vi "Store Active Guidance.vi"(8 "error in (no error)":errorcluster, 10 "Guidance In":refnum<class "Guidance.lvclass">, 11 "Vessel in":refnum<class "Vessel.lvclass">) -> (0 "error out":errorcluster, 3 "Vessel out":refnum<class "Vessel.lvclass">)   [LabVIEW 2014, in "Vessel.lvclass"]
uses:
  Vessel.lvclass
  Guidance/Guidance.lvclass
  Vessel.lvclass/Vessel.ctl
  Supervisor/Supervisor.lvclass
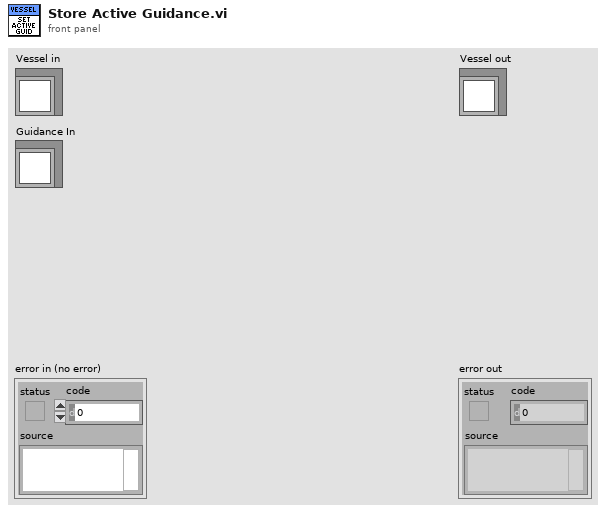
[diagram p1: front panel]
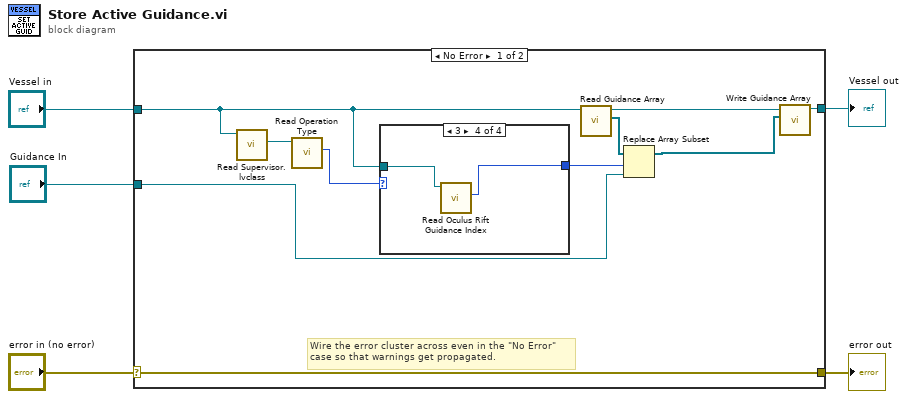
[diagram p0: block diagram]
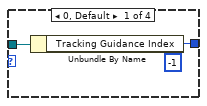
[diagram p2: hidden frame]
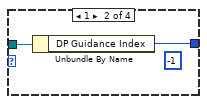
[diagram p3: hidden frame]
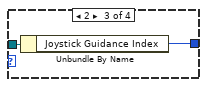
[diagram p4: hidden frame]
diagram:
  n1 = case shown="No Error" "error in (no error)" {
    selector: "error in (no error)" -> [w15 w25]
    tunnel: [w15 w25] -> w4
    tunnel: [w10 w24] -> w2
    tunnel: "Vessel in" -> [w11 w24]
    tunnel: "Guidance In" -> [w7 _]
    frame No Error {
      # "Wire the error cluster across even in the \"No Error\"\ncase so that warnings get propagated."
      n2 = call "Read Supervisor.lvclass.vi"("Vessel in"=w11) -> ("Supervisor.lvclass"=w14:refnum<class "Supervisor.lvclass">)  [unwired: 8 in, 2 out]
      n3 = call-dynamic "Read Operation Type.vi"("Supervisor in"=w14) -> ("Operation Type"=w13:u16)  [unwired: 8 in, 2 out]
      n4 = case shown="3" w13 {
        tunnel: w11 -> [w17 w19 w21 w23]
        tunnel: [w16 w18 w20 w22] -> w8
        frame 0, Default {
          (unwired) -1 ("DP Guidance Index")
          n5 = Unbundle By Name(w17) -> ("Tracking Guidance Index"=w16:i32)
        }
        frame 1 {
          (unwired) -1 ("DP Guidance Index")
          n6 = Unbundle By Name(w19) -> ("DP Guidance Index"=w18:i32)
        }
        frame 2 {
          n7 = Unbundle By Name(w21) -> ("Joystick Guidance Index"=w20:i32)
        }
        frame 3 {
          n8 = call-dynamic "Read Oculus Rift Guidance Index.vi"("Vessel in"=w23) -> ("Oculus Rift Guidance Index"=w22:i32)  [unwired: 8 in, 2 out]
        }
      }
      n9 = call "Read Guidance Array.vi"("Vessel in"=w11) -> ("Guidance Array"=w9:refnum<class "Guidance.lvclass">[], "Vessel out"=w12:refnum<class "Vessel.lvclass">)  [unwired: 8 in, 1 out]
      n10 = Replace Array Subset(array=w9, new element=w7, index=w8) -> (w6:refnum<class "Guidance.lvclass">[])
      n11 = call "Write Guidance Array.vi"("Guidance Array"=w6, "Vessel in"=w12) -> ("Vessel out"=w10:refnum<class "Vessel.lvclass">)  [unwired: 8 in, 1 out]
    }
    frame Error {
    }
  }
  "error out" <- w4
  "Vessel out" <- w2
